vi "getRegisters.vi"(0 "AddressSpace in":refnum<class "AddressSpace.lvclass">) -> (4 "AddressSpace out":refnum<class "AddressSpace.lvclass">, 8 "Parameters":T1={"Deadtime"="Deadtime", "Period"="Period", "A_timing"="A_timing", "B_timing"="B_timing", "C_timing"="C_timing"})   [LabVIEW 2017, in "SVPWM.lvlib" / "AddressSpace.lvclass"]
uses:
  AddressSpace.lvclass
  Parameters.ctl
  AddressSpace.lvclass/AddressSpace.ctl
  SVPWM.lvlib
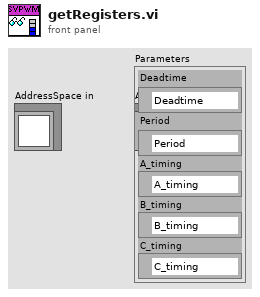
[diagram p1: front panel]
types:
  T1 = typedef "SVPWM.lvlib/Parameters.ctl" = cluster{"Deadtime":refnum<k21>, "Period":refnum<k21>, "A_timing":refnum<k21>, "B_timing":refnum<k21>, "C_timing":refnum<k21>}
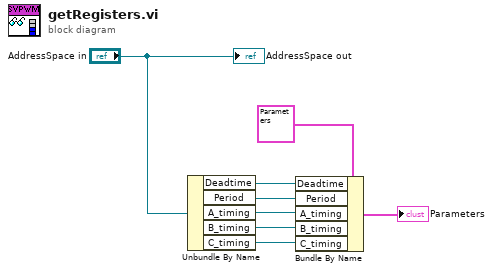
[diagram p0: block diagram]
diagram:
  n1 = Unbundle By Name("AddressSpace in") -> ("Deadtime"=w5:refnum<k21>, "Period"=w6:refnum<k21>, "A_timing"=w3:refnum<k21>, "B_timing"=w2:refnum<k21>, "C_timing"=w1:refnum<k21>)
  n2 = Bundle By Name(cluster=T1 {"Deadtime"="Deadtime", "Period"="Period", "A_timing"="A_timing", "B_timing"="B_timing", "C_timing"="C_timing"} ("Parameters"), "Deadtime"=w5, "Period"=w6, "A_timing"=w3, "B_timing"=w2, "C_timing"=w1) -> (→"Parameters":T1)
  "AddressSpace out" <- "AddressSpace in"
